vi "RSZVB Send Channel Trigger.vi"(8 "error in (no error)":errorcluster {"code" format="%.0x"}, 10 "Channel (1)":i32=1, 11 "VISA session":refnum<visa-resource-name>) -> (0 "error out":errorcluster {"code" format="%.0x"}, 3 "dup VISA session":refnum<visa-resource-name>)   [LabVIEW 2011]
doc: "This VI starts a new single sweep sequence. This VI is available in single sweep mode only (INITiate<Ch>:CONTinuous OFF).\n\nNote(s):\n\n(1) In contrast to all other functions of the analyzer, INITiate<Ch>[:IMMediate] has been implemented to prevent overlapped execution.\n\n(2) The data of the last sweep can be read using CALCulate<Ch>:DATA:NSWeep? SDATa, <history_count>.\n\nRemote-control command(s):\nINITiate<Ch>[:IMMediate]"
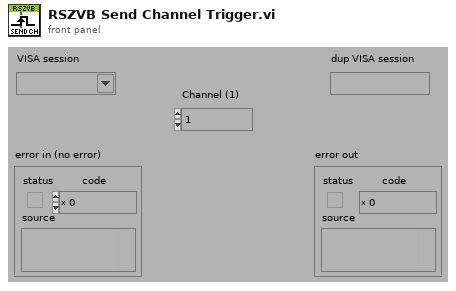
[diagram p1: front panel]
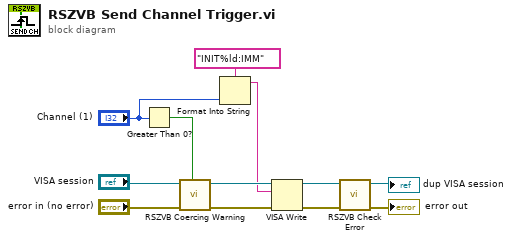
[diagram p0: block diagram]
diagram:
  n1 = Greater Than 0?(x="Channel (1)") -> (x > 0?=w11:bool)
  n2 = call "RSZVB Coercing Warning.vi"("In Range?"=w11, "error in (no error)"="error in (no error)", "VISA session"="VISA session") -> ("error out"=w8:errorcluster, "dup VISA session"=w9:refnum<visa-resource-name>)  [unwired: 7 in]
  n3 = Format Into String(format string="INIT%ld:IMM", "Channel (1)") -> (resulting string=w3:string)  [unwired: 2 in, 1 out]
  n4 = VISA Write(VISA resource name=w9, write buffer=w3, error in (no error)=w8) -> (VISA resource name out=w6:refnum<visa-resource-name>, error out=w7:errorcluster)  [unwired: 1 out]
  n5 = call "RSZVB Check Error.vi"("error in (no error)"=w7, "VISA session"=w6) -> ("error out"=→"error out":errorcluster, "dup VISA session"=→"dup VISA session":refnum<visa-resource-name>)  [unwired: 8 in]
